vi "Remote AQ Module.vi"(6 "error in":errorcluster, 9 "device ID":refnum<k1>) -> (0 "error out":errorcluster, 1 "Claw Motor":u32(slide) scale=0.0..100.0, 2 "Elbow Motor":u32(slide)=50 scale=0.0..100.0, 3 "device ID 2":refnum<k1>, 4 "Boolean":T1, 5 "Direction":T2, 7 "Shoulder Motor":u32(slide)=50 scale=0.0..100.0, 8 "Base Motor":u32(slide)=50 scale=0.0..100.0)   [LabVIEW 2015]
uses:
  DIR GAME.ctl
  GAME CLUST.ctl
  <vilib>/Utility/inputDevices.llb/joystickAcquire.vi
panel:
  # "Arm Controls"
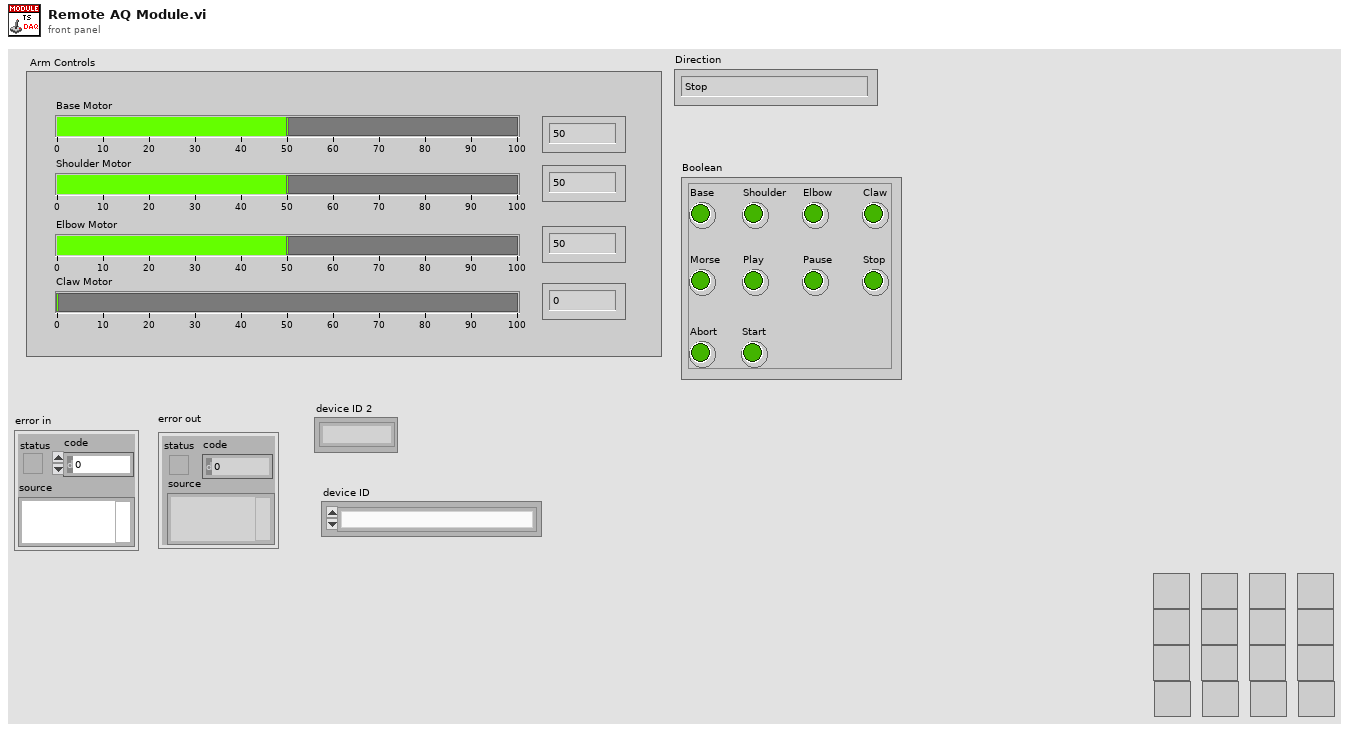
[diagram p1: front panel]
types:
  T1 = typedef "GAME CLUST.ctl" = cluster{"Base":bool, "Shoulder":bool, "Elbow":bool, "Claw":bool, "Morse":bool, "Play":bool, "Pause":bool, "Stop":bool, "Abort":bool, "Start":bool}
  T2 = typedef "DIR GAME.ctl" = enum16{"Stop", "Front", "FR", "Right", "BR", "Back", "BL", "Left", "FL"}
  T3 = cluster{"Base":bool, "Shoulder":bool, "Elbow":bool, "Claw":bool, "Morse":bool, "Play":bool, "Pause":bool, "Stop":bool, "Abort":bool, "Start":bool}
  T4 = cluster{"X axis":i32, "Y axis":i32, "Z axis":i32, "X axis rotation":i32, "Y axis rotation":i32, "Z axis rotation":i32, "U axis":i32, "V axis":i32}
  T5 = cluster{"button 1":bool, "button 2":bool, "button 3":bool, "button 4":bool, "button 5":bool, "button 6":bool, "button 7":bool, "button 8":bool, "button 9":bool, "button 10":bool, "button 11":bool, "button 12":bool, "button 13":bool, "button 14":bool, "button 15":bool, "button 16":bool, "button 17":bool, "button 18":bool, "button 19":bool, "button 20":bool, "button 21":bool, "button 22":bool, "button 23":bool, "button 24":bool, "button 25":bool, "button 26":bool, "button 27":bool, "button 28":bool, "button 29":bool, "button 30":bool, "button 31":bool, "button 32":bool}
  T6 = cluster{"pov 1":i32, "pov 2":i32, "pov 3":i32, "pov 4":i32}
  T7 = enum16{"Stop", "Front", "FR", "Right", "BR", "Back", "BL", "Left", "FL"}
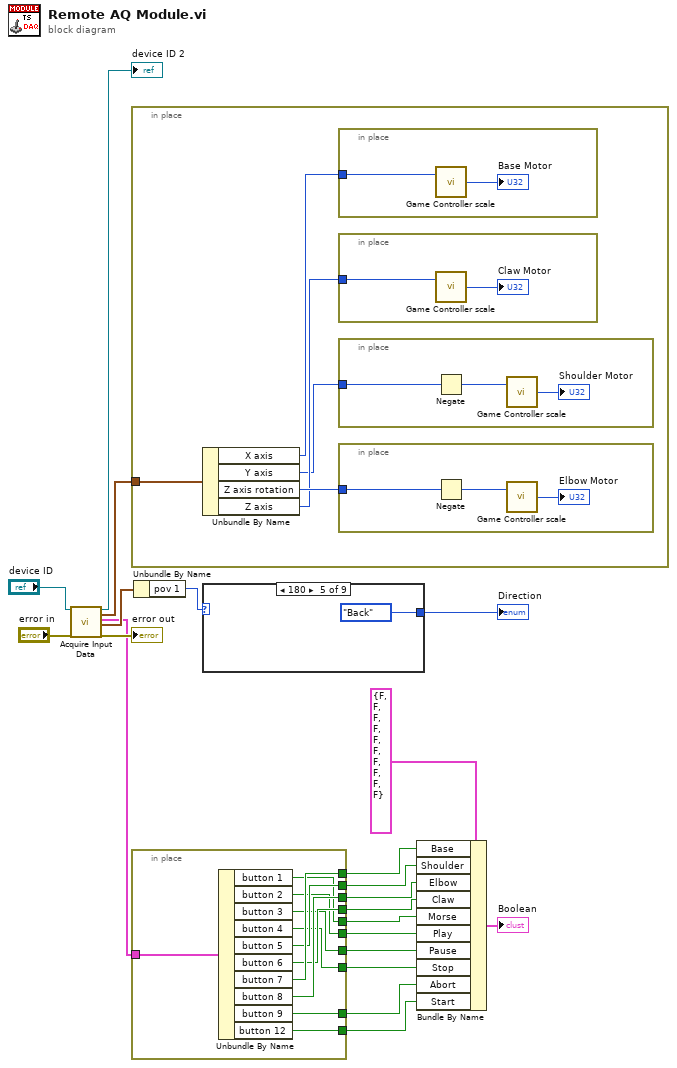
[diagram p0: block diagram]
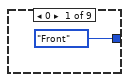
[diagram p2: hidden frame]
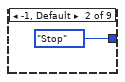
[diagram p3: hidden frame]
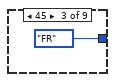
[diagram p4: hidden frame]
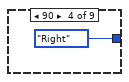
[diagram p5: hidden frame]
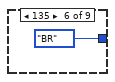
[diagram p6: hidden frame]
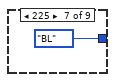
[diagram p7: hidden frame]
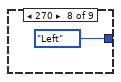
[diagram p8: hidden frame]
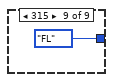
[diagram p9: hidden frame]
diagram:
  n1 = call-poly <vilib>:"Acquire Input Data.vi"("device ID"="device ID", "error in (no error)"="error in") -> ("device ID"=→"device ID 2":refnum<k1>, "axis info"=w12:T4, "button info"=w11:T5, "direction info"=w13:T6, "error out"=→"error out":errorcluster)  [unwired: 13 in]
  n2 = in-place {
    in-place-border: w12 -> [w26]
    n3 = Unbundle By Name(w26) -> ("X axis"=w25:i32, "Y axis"=w22:i32, "Z axis rotation"=w24:i32, "Z axis"=w23:i32)
    n4 = in-place {
      in-place-border: w25 -> [w32]
      n5 = call "Game Controller scale.vi"("Game controller in"=w32) -> ("Arm out"=→"Base Motor":u32)  [unwired: 1 in]
    }
    n6 = in-place {
      in-place-border: w23 -> [w27]
      n7 = call "Game Controller scale.vi"("Game controller in"=w27) -> ("Arm out"=→"Claw Motor":u32)  [unwired: 1 in]
    }
    n8 = in-place {
      in-place-border: w22 -> [w36]
      n9 = Negate(x=w36) -> (-x=w35:i32)
      n10 = call "Game Controller scale.vi"("Game controller in"=w35) -> ("Arm out"=→"Shoulder Motor":u32)  [unwired: 1 in]
    }
    n11 = in-place {
      in-place-border: w24 -> [w30]
      n12 = Negate(x=w30) -> (-x=w29:i32)
      n13 = call "Game Controller scale.vi"("Game controller in"=w29) -> ("Arm out"=→"Elbow Motor":u32)  [unwired: 1 in]
    }
  }
  n14 = in-place {
    in-place-border: w11 -> [w47]
    in-place-border: [w46] -> w10
    in-place-border: [w45] -> w9
    in-place-border: [w44] -> w8
    in-place-border: [w43] -> w7
    in-place-border: [w42] -> w6
    in-place-border: [w41] -> w5
    in-place-border: [w40] -> w4
    in-place-border: [w39] -> w3
    in-place-border: [w38] -> w20
    in-place-border: [w37] -> w19
    n15 = Unbundle By Name(w47) -> ("button 1"=w42:bool, "button 2"=w41:bool, "button 3"=w40:bool, "button 4"=w39:bool, "button 5"=w45:bool, "button 6"=w43:bool, "button 7"=w46:bool, "button 8"=w44:bool, "button 9"=w37:bool, "button 12"=w38:bool)
  }
  n16 = Unbundle By Name(w13) -> ("pov 1"=w14:i32)
  n17 = case shown="180" w14 {
    tunnel: [T7."Front" ("Enum 2") T7."Stop" ("Enum 2") T7."FR" ("Enum 2") T7."Right" ("Enum 2") T7."Back" ("Enum 2") T7."BR" ("Enum 2") T7."BL" ("Enum 2") T7."Left" ("Enum 2") T7."FL" ("Enum 2")] -> w15
    frame 0 {
    }
    frame -1, Default {
    }
    frame 45 {
    }
    frame 90 {
    }
    frame 180 {
    }
    frame 135 {
    }
    frame 225 {
    }
    frame 270 {
    }
    frame 315 {
    }
  }
  "Direction" <- w15
  n18 = Bundle By Name(cluster=T3 {"Base"=FALSE, "Shoulder"=FALSE, "Elbow"=FALSE, "Claw"=FALSE, "Morse"=FALSE, "Play"=FALSE, "Pause"=FALSE, "Stop"=FALSE, "Abort"=FALSE, "Start"=FALSE} ("Boolean 2"), "Base"=w10, "Shoulder"=w9, "Elbow"=w8, "Claw"=w7, "Morse"=w6, "Play"=w5, "Pause"=w4, "Stop"=w3, "Abort"=w19, "Start"=w20) -> (→"Boolean":T3)
